vi "pwm_control.vi"() -> (0 "error out":errorcluster)   [LabVIEW 2013]
panel:
  in  "pwm info":T1
  out "status":string
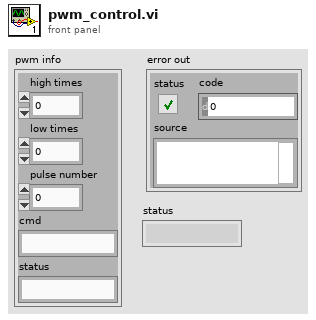
[diagram p1: front panel]
types:
  T1 = cluster{"high times":dbl, "low times":dbl, "pulse number":i32, "cmd":string, "status":string}
  T2 = cluster{"sample mode":i32, "initial delay":dbl, "idle state":i32, "counter":string, "channel name":string, "low time":dbl, "high time":dbl, "units":i32, "number of samples":i32}
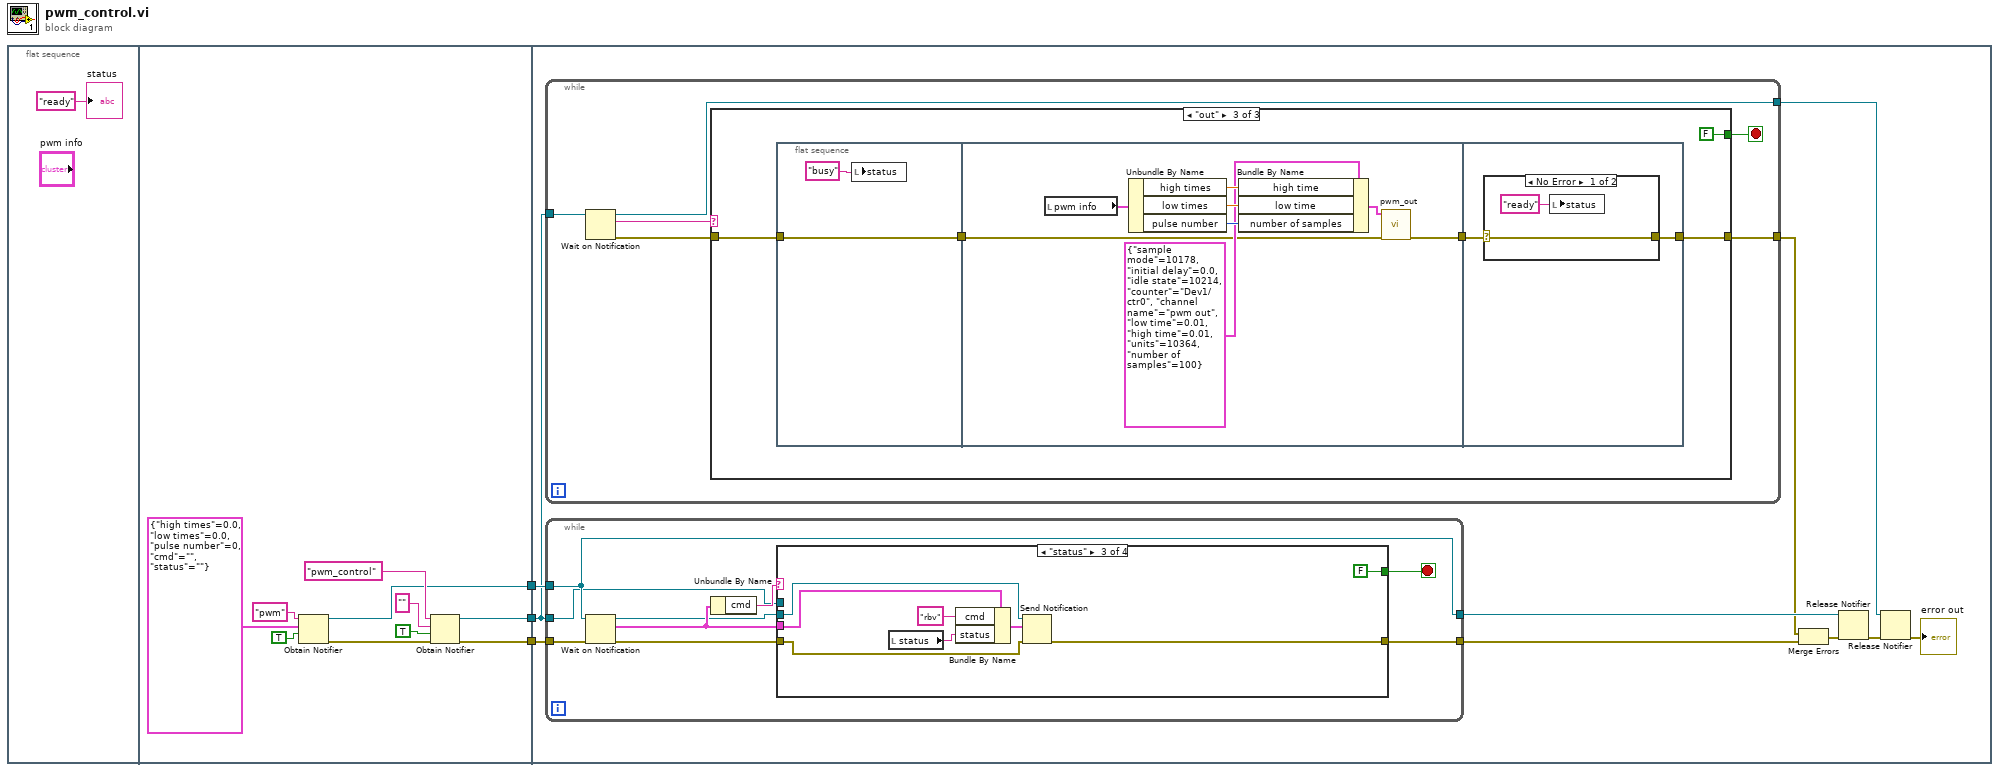
[diagram p0: block diagram]
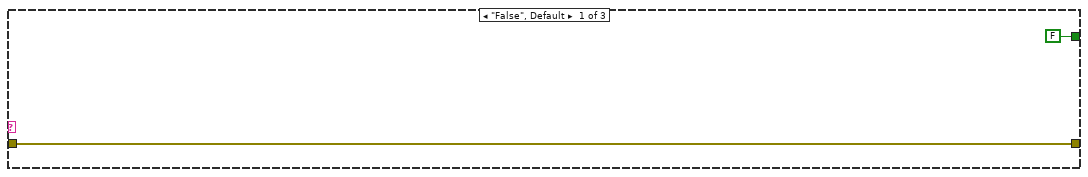
[diagram p2: hidden frame]
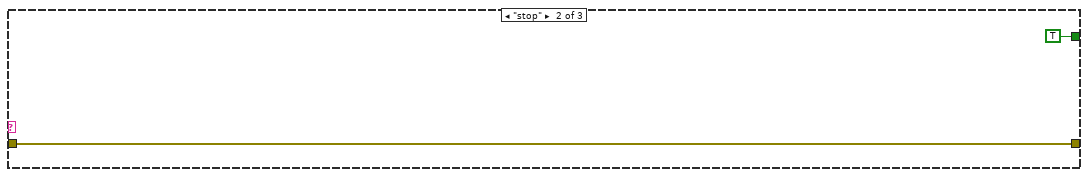
[diagram p3: hidden frame]
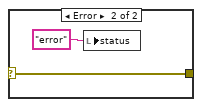
[diagram p4: hidden frame]
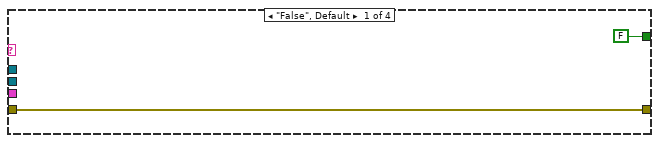
[diagram p5: hidden frame]
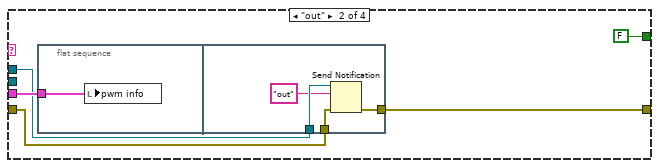
[diagram p6: hidden frame]
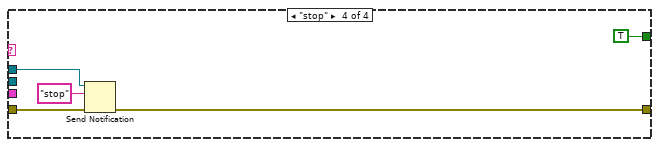
[diagram p7: hidden frame]
diagram:
  n1 = flat-sequence {
    tunnel: [w6] -> w3
    tunnel: [w12] -> w2
    tunnel: [w11] -> w1
    tunnel: w3 -> [w24]
    tunnel: w2 -> [w23]
    tunnel: w1 -> [w22]
    frame #0 {
      "status" <- "ready"
    }
    frame #1 {
      n2 = Obtain Notifier(name (unnamed)="pwm", notification data type=T1 {"high times"=0.0, "low times"=0.0, "pulse number"=0, "cmd"="", "status"=""}, create if not found? (T)=TRUE) -> (notifier out=w6:refnum<notifier>, error out=w5:errorcluster)  [unwired: 1 in, 1 out]
      n3 = Obtain Notifier(name (unnamed)="pwm_control", notification data type="", create if not found? (T)=TRUE, error in (no error)=w5) -> (notifier out=w11:refnum<notifier>, error out=w12:errorcluster)  [unwired: 1 out]
    }
    frame #2 {
      n4 = while {
        tunnel: w22 -> [w30]
        tunnel: [w26] -> w21
        tunnel: [w25] -> w18
        stop <- w28 stop-if-true
        n5 = Wait on Notification(notifier=w30) -> (notifier out=w26:refnum<notifier>, notification=w29:string, error out=w27:errorcluster)  [unwired: 3 in, 1 out]
        n6 = case shown="\"out\"" w29 {
          tunnel: [FALSE TRUE FALSE] -> w28
          tunnel: w27 -> [w31 w33 w37]
          tunnel: [w31 w33 w35] -> w25
          frame "False", Default {
          }
          frame "stop" {
          }
          frame "out" {
            n7 = flat-sequence {
              tunnel: w37 -> [w40]
              tunnel: [w40] -> w36
              tunnel: [w43] -> w39
              tunnel: w36 -> [w42]
              tunnel: w39 -> [w51]
              tunnel: [w50] -> w35
              frame #0 {
                n8 = local write "status"("busy") -> ()
              }
              frame #1 {
                n9 = local read "pwm info"() -> (w46:T1)
                n10 = Unbundle By Name(w46) -> ("high times"=w47:dbl, "low times"=w48:dbl, "pulse number"=w49:i32)
                n11 = Bundle By Name(cluster=T2 {"sample mode"=10178, "initial delay"=0.0, "idle state"=10214, "counter"="Dev1/ctr0", "channel name"="pwm out", "low time"=0.01, "high time"=0.01, "units"=10364, "number of samples"=100} ("pwm info"), "high time"=w47, "low time"=w48, "number of samples"=w49) -> (w44:T2)
                n12 = call "pwm_out.vi"("pwm info"=w44, "error in"=w42) -> ("error out"=w43:errorcluster)  [unwired: 13 in]
              }
              frame #2 {
                n13 = case shown="No Error" w51 {
                  selector: w51 -> [w52 w54]
                  tunnel: [w52 w54] -> w50
                  frame No Error {
                    n14 = local write "status"("ready") -> ()
                  }
                  frame Error {
                    n15 = local write "status"("error") -> ()
                  }
                }
              }
            }
          }
        }
      }
      n16 = while {
        tunnel: [w61] -> w20
        tunnel: w24 -> [w61]
        tunnel: w23 -> [w60]
        tunnel: w22 -> [w59]
        tunnel: [w56] -> w17
        stop <- w63 stop-if-true
        n17 = Wait on Notification(notifier=w61, error in (no error)=w60) -> (notifier out=w58:refnum<notifier>, notification=w62:T1, error out=w57:errorcluster)  [unwired: 2 in, 1 out]
        n18 = Unbundle By Name(w62) -> ("cmd"=w64:string)
        n19 = case shown="\"status\"" w64 {
          tunnel: [FALSE FALSE FALSE TRUE] -> w63
          tunnel: w62 -> [_ w70 w83 _]
          tunnel: w59 -> [_ w69 _ w88]
          tunnel: w58 -> [_ _ w84 _]
          tunnel: w57 -> [w65 w68 w78 w86]
          tunnel: [w65 w67 w77 w85] -> w56
          frame "False", Default {
          }
          frame "out" {
            n20 = flat-sequence {
              tunnel: w70 -> [w72]
              tunnel: w69 -> [w76]
              tunnel: w68 -> [w74]
              tunnel: [w73] -> w67
              frame #0 {
                n21 = local write "pwm info"(w72) -> ()
              }
              frame #1 {
                n22 = Send Notification(notification="out", notifier=w76, error in (no error)=w74) -> (error out=w73:errorcluster)  [unwired: 1 out]
              }
            }
          }
          frame "status" {
            n23 = local read "status"() -> (w81:string)
            n24 = Bundle By Name(cluster=w83, "cmd"="rbv", "status"=w81) -> (w80:T1)
            n25 = Send Notification(notification=w80, notifier=w84, error in (no error)=w78) -> (error out=w77:errorcluster)  [unwired: 1 out]
          }
          frame "stop" {
            n26 = Send Notification(notification="stop", notifier=w88, error in (no error)=w86) -> (error out=w85:errorcluster)  [unwired: 1 out]
          }
        }
      }
      n27 = Merge Errors(w18, w17) -> (w16:errorcluster)
      n28 = Release Notifier(notifier=w20, error in (no error)=w16) -> (error out=w19:errorcluster)  [unwired: 1 in, 2 out]
      n29 = Release Notifier(notifier=w21, error in (no error)=w19) -> (error out=→"error out":errorcluster)  [unwired: 1 in, 2 out]
    }
  }
